vi "test_Util_All.vi"(8 "error in (no error)":errorcluster) -> (0 "error out":errorcluster, 3 "Test Passed":bool)   [LabVIEW 2019]
panel:
  out "Xform Test Passed":bool
  out "Dist Test Passed":bool
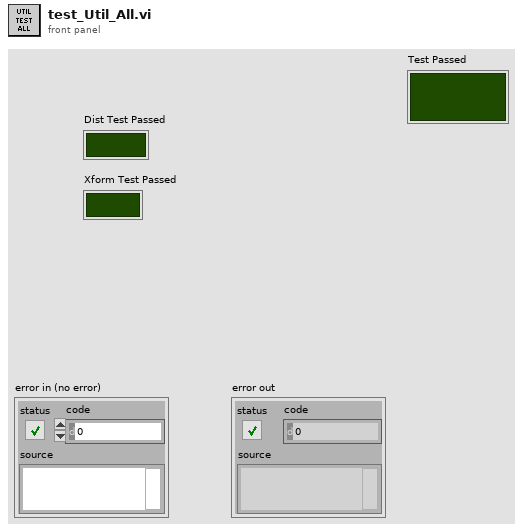
[diagram p1: front panel]
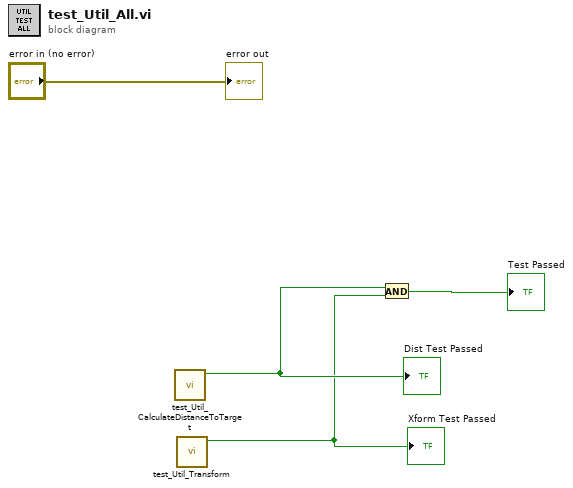
[diagram p0: block diagram]
diagram:
  n1 = call "test_Util_CalculateDistanceToTarget.vi"() -> ("Test Passed"=w2:bool)  [unwired: 10 in, 1 out]
  "Dist Test Passed" <- w2
  n2 = call "test_Util_Transform.vi"() -> ("Test Passed"=w1:bool)  [unwired: 10 in, 1 out]
  "Xform Test Passed" <- w1
  n3 = And(x=w2, y=w1) -> (x .and. y?=→"Test Passed":bool)
  "error out" <- "error in (no error)"
